vi "KE622x -- Set Trig Bypass State.vi"(0 "Resource In":refnum<visa-resource-name>, 1 "Check For SCPI Errors? (T)":bool=TRUE, 7 "Bypass Trig Layer?":bool, 11 "error in (no error)":errorcluster) -> (4 "Resource Out (dupl)":refnum<visa-resource-name>, 15 "error out":errorcluster)   [LabVIEW 2019, in "Keithley 622x.lvlib"]
uses:
  Keithley 622x.lvlib
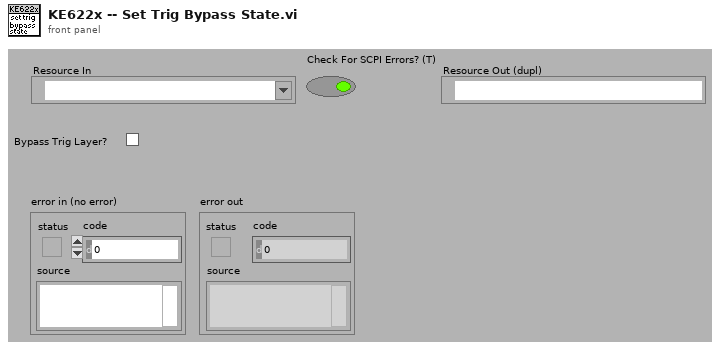
[diagram p1: front panel]
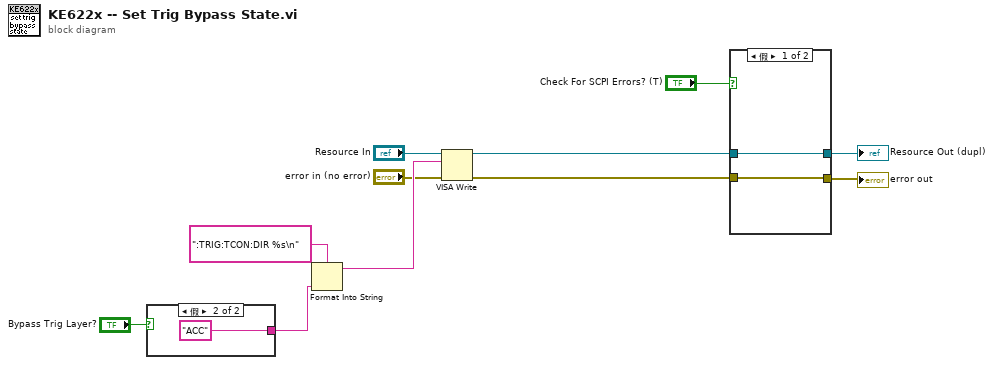
[diagram p0: block diagram]
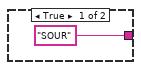
[diagram p2: hidden frame]
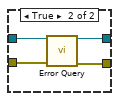
[diagram p3: hidden frame]
diagram:
  n1 = case shown="假" "Bypass Trig Layer?" {
    tunnel: ["SOUR" "ACC"] -> w3
    frame True {
    }
    frame False {
    }
  }
  n2 = Format Into String(format string=":TRIG:TCON:DIR %s\n", w3) -> (resulting string=w9:string)  [unwired: 2 in, 1 out]
  n3 = VISA Write(VISA resource name="Resource In", write buffer=w9, error in (no error)="error in (no error)") -> (VISA resource name out=w6:refnum<visa-resource-name>, error out=w5:errorcluster)  [unwired: 1 out]
  n4 = case shown="假" "Check For SCPI Errors? (T)" {
    tunnel: w6 -> [w15 w19]
    tunnel: w5 -> [w14 w18]
    tunnel: [w14 w17] -> w1
    tunnel: [w15 w16] -> w2
    frame False {
    }
    frame True {
      n5 = call "Error Query.vi"("VISA Resource In"=w19, "error in (no error)"=w18) -> ("VISA Resource Out (dupl)"=w16:refnum<visa-resource-name>, "error out"=w17:errorcluster)  [unwired: 10 in, 2 out]
    }
  }
  "Resource Out (dupl)" <- w2
  "error out" <- w1
